vi "ENC RT.vi"(8 "错误输入（无错误）":errorcluster, 10 "Reset ENC":bool, 11 "Custom FPGA Reference Out":refnum<k20>) -> (0 "错误输出":errorcluster, 2 "ENC":i32[](array[numeric]), 3 "FPGA VI引用输出":refnum<k20>)   [LabVIEW 2017]
uses:
  <vilib>/Utility/error.llb/Error Cluster From Error Code.vi
  <vilib>/rvi/errors/niLvFpgaAdjustHostInterfaceError.vi
  <vilib>/rvi/interface/nirviReadWriteControl/nirviReadWriteControl.xnode
  <vilib>/rvi/interface/Simulation/niFpgaSimulationCallBeginRW.vi
  NiFpgaLv.dll
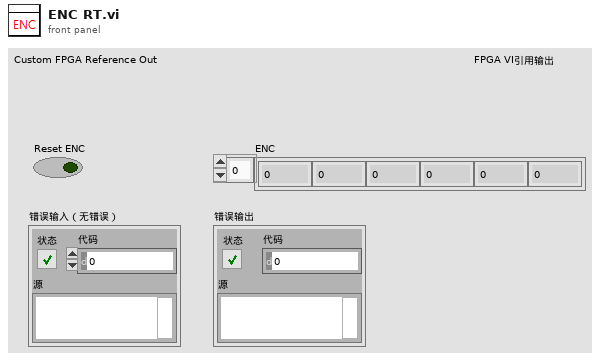
[diagram p1: front panel]
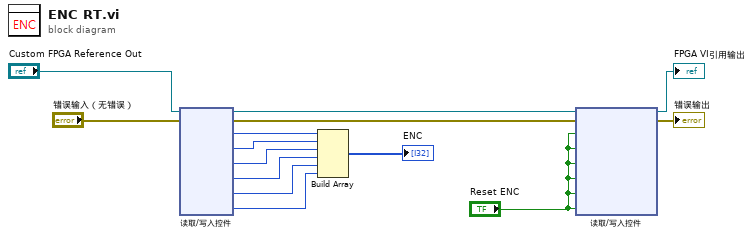
[diagram p0: block diagram]
diagram:
  n1 = xnode "读取/写入控件"("FPGA VI引用输入"="Custom FPGA Reference Out", "错误输入"="错误输入（无错误）") -> ("FPGA VI引用输出"=w3:refnum<k20>, "错误输出"=w12:errorcluster, "ENC 1"=w5:i32, "ENC 2"=w6:i32, "ENC 3"=w7:i32, "ENC 6"=w8:i32, "ENC 4"=w9:i32, "ENC 5"=w10:i32)
  n2 = Build Array(w5, w6, w7, w8, w9, w10) -> (→"ENC":i32[])
  n3 = xnode "读取/写入控件"("FPGA VI引用输入"=w3, "错误输入"=w12, "Reset ENC 1"="Reset ENC", "Reset ENC 2"="Reset ENC", "Reset ENC 3"="Reset ENC", "Reset ENC 4"="Reset ENC", "Reset ENC 5"="Reset ENC", "Reset ENC 6"="Reset ENC") -> ("FPGA VI引用输出"=→"FPGA VI引用输出":refnum<k20>, "错误输出"=→"错误输出":errorcluster)
